vi "DWE Decode Data.vi"(8 "Errors In":T1, 9 "Prev time stamp":timestamp, 10 "Time Stamp":timestamp, 11 "Data Array":string[](array[string])) -> (0 "Errors Out":T1, 3 "logData Out":T2)   [LabVIEW 2014]
doc: "Decode hex data obtained from inverter boards into decimal measurements. DC bus voltage, current RMS, motor power, temp."
uses:
  TypeDefs/DWE Errors.ctl
panel:
  out "Elapsed time (min)":dbl
  out "Elapsed time (sec)":dbl
  in  "logData In":T3
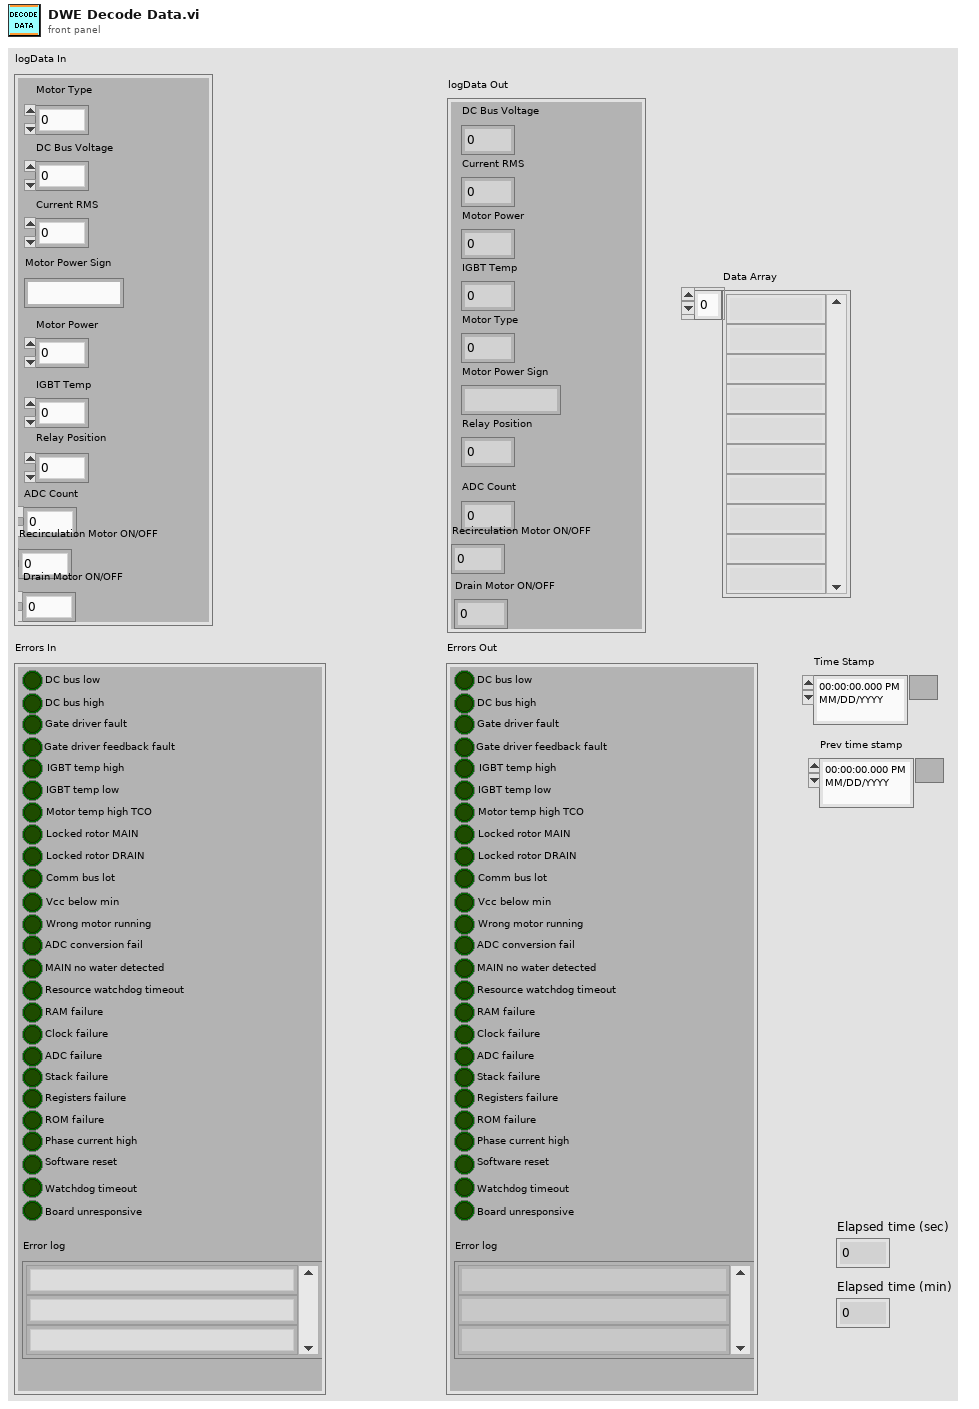
[diagram p1: front panel]
types:
  T1 = typedef "DWE Errors.ctl" = cluster{"DC bus low":bool, "DC bus high":bool, "Gate driver fault":bool, "Gate driver feedback fault":bool, "IGBT temp high":bool, "IGBT temp low":bool, "Motor temp high TCO":bool, "Locked rotor MAIN":bool, "Locked rotor DRAIN":bool, "Comm bus lot":bool, "Vcc below min":bool, "Wrong motor running":bool, "ADC conversion fail":bool, "MAIN no water detected":bool, "Resource watchdog timeout":bool, "RAM failure":bool, "Clock failure":bool, "ADC failure":bool, "Stack failure":bool, "Registers failure":bool, "ROM failure":bool, "Phase current high":bool, "Software reset":bool, "Watchdog timeout":bool, "Error log":string[], "Board unresponsive":bool}
  T2 = cluster{"DC Bus Voltage":dbl, "Current RMS":dbl, "Motor Power":dbl, "IGBT Temp":u16, "Motor Type":u16, "Motor Power Sign":string, "Relay Position":u16, "ADC Count":dbl, "Recirculation Motor ON/OFF":u16, "Drain Motor ON/OFF":u16}
  T3 = cluster{"DC Bus Voltage":dbl, "Current RMS":dbl, "Motor Power":dbl, "IGBT Temp":u32, "Motor Type":u16, "Motor Power Sign":string, "Relay Position":u16, "ADC Count":dbl, "Recirculation Motor ON/OFF":u32, "Drain Motor ON/OFF":u16}
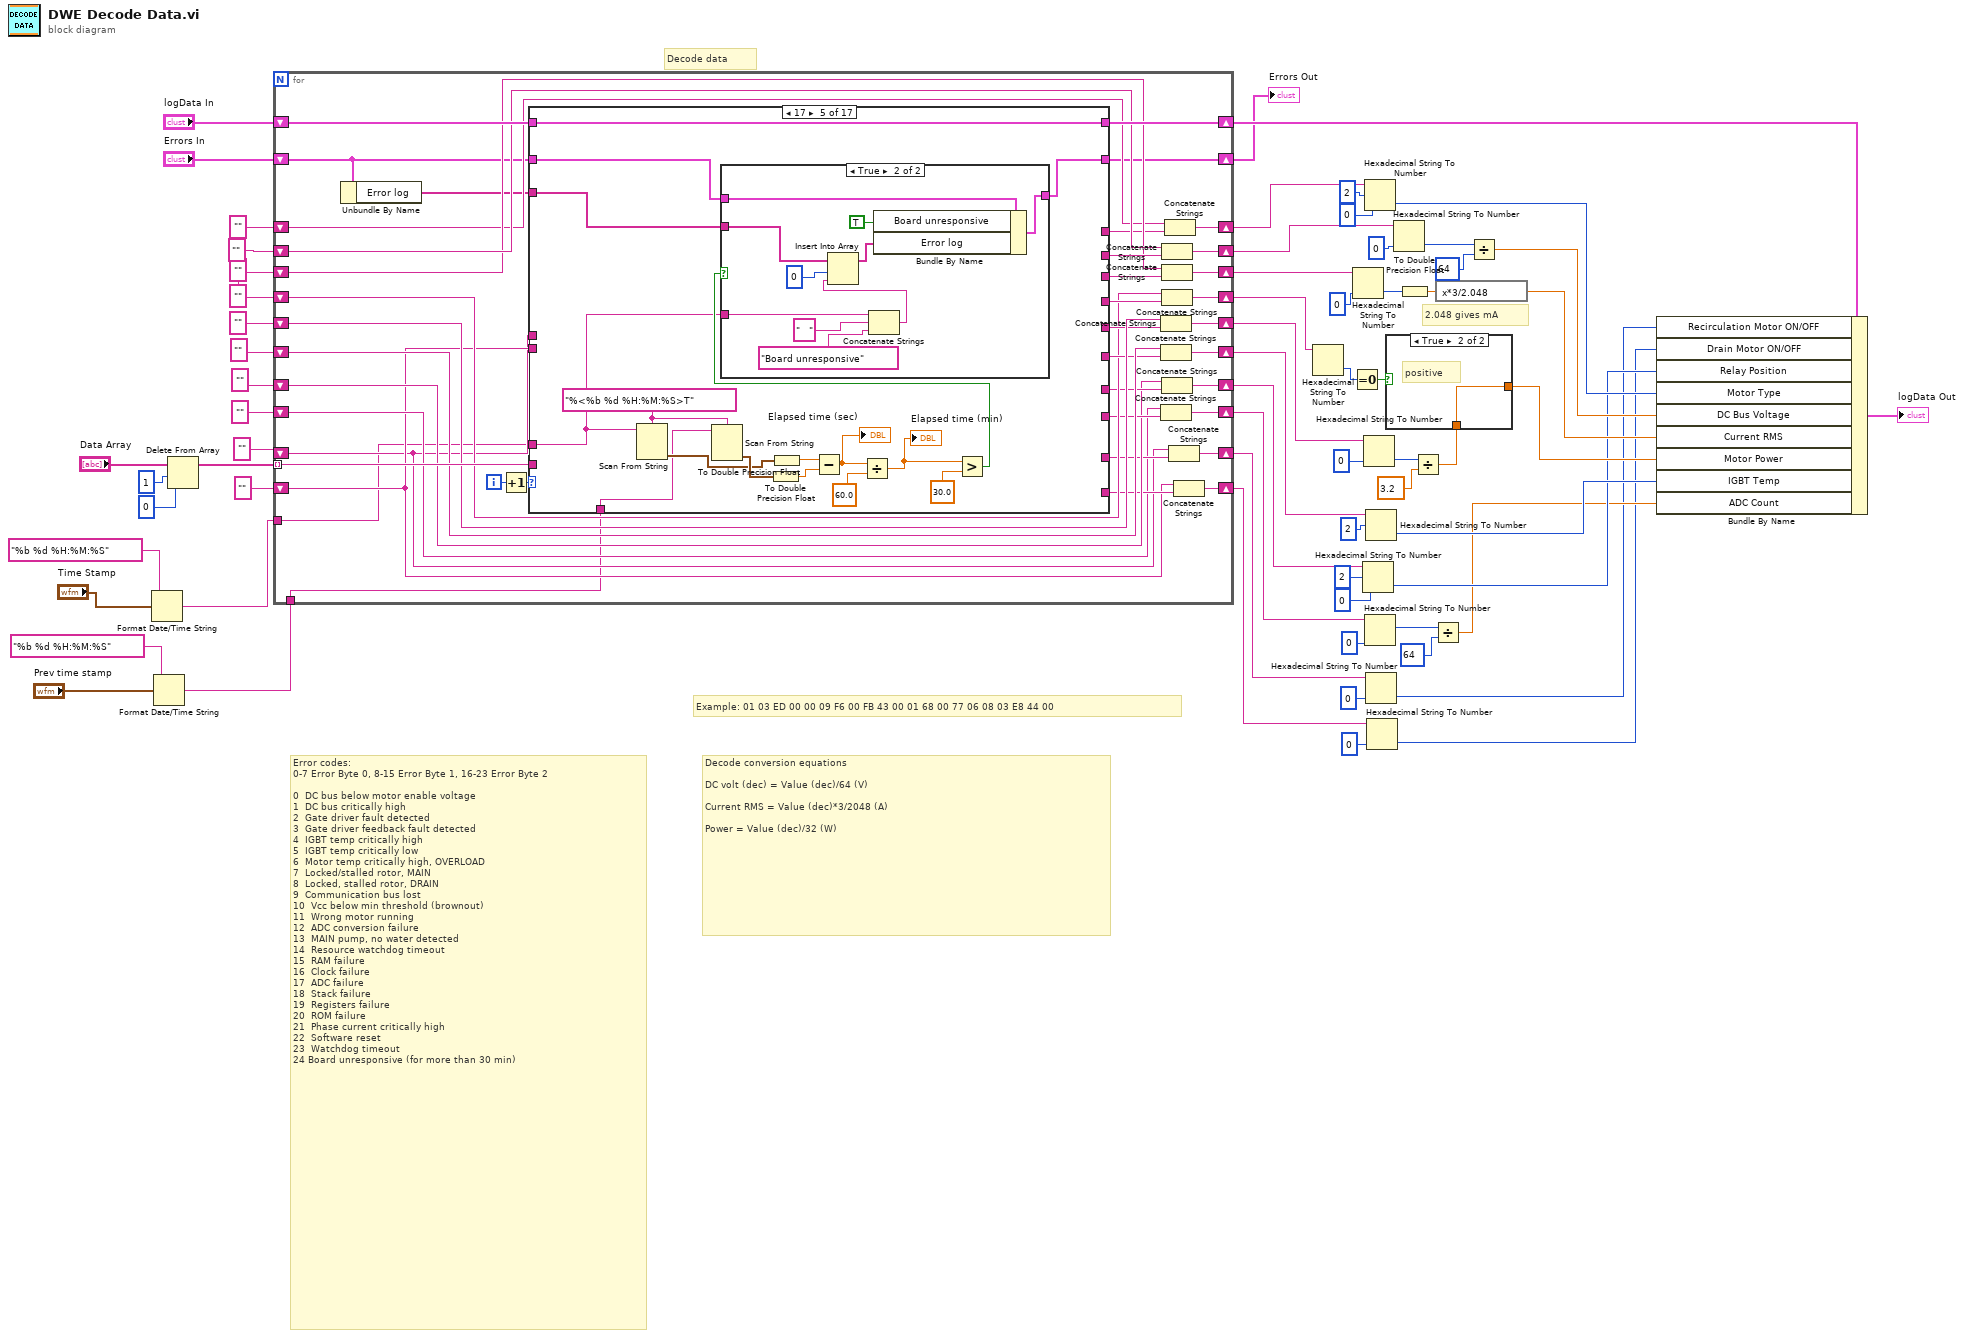
[diagram p0: block diagram]
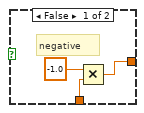
[diagram p2: hidden frame]
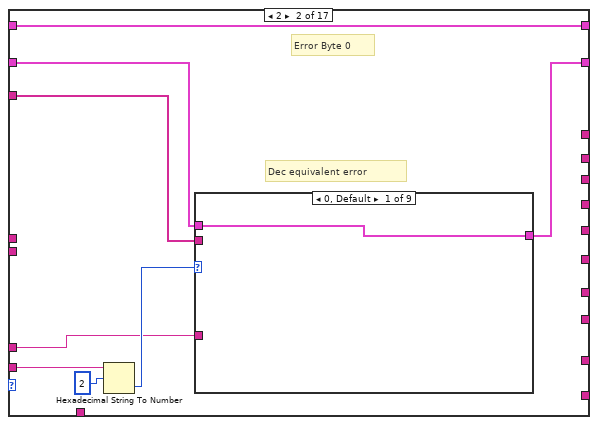
[diagram p4: hidden frame]
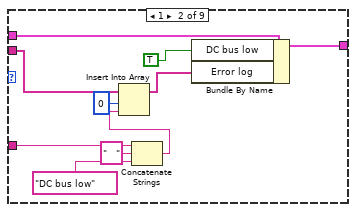
[diagram p5: hidden frame]
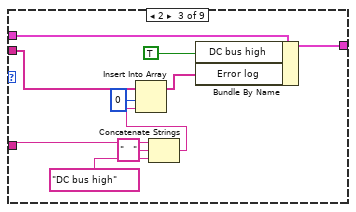
[diagram p6: hidden frame]
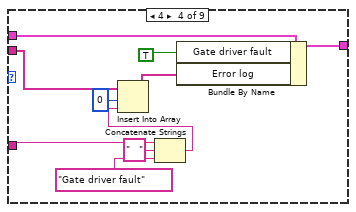
[diagram p7: hidden frame]
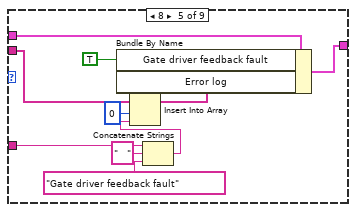
[diagram p8: hidden frame]
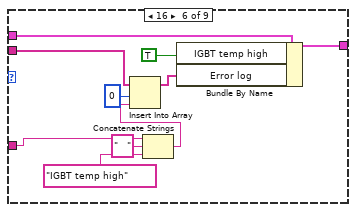
[diagram p9: hidden frame]
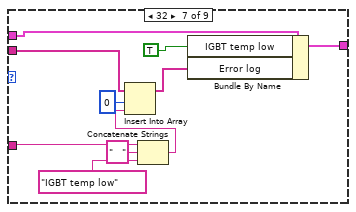
[diagram p10: hidden frame]
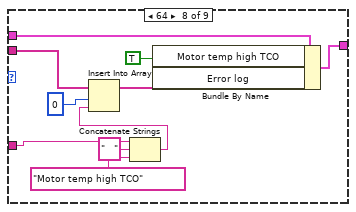
[diagram p11: hidden frame]
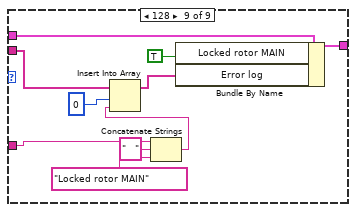
[diagram p12: hidden frame]
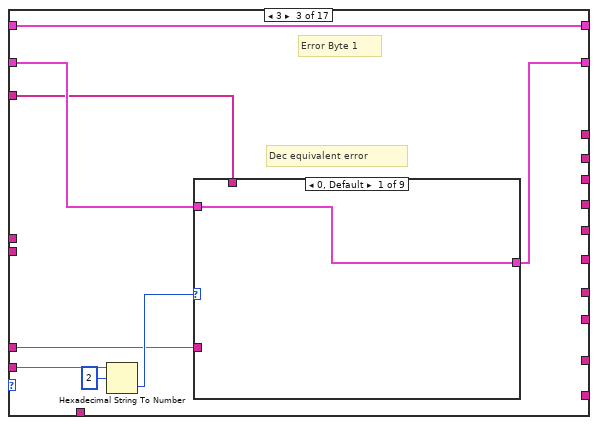
[diagram p13: hidden frame]
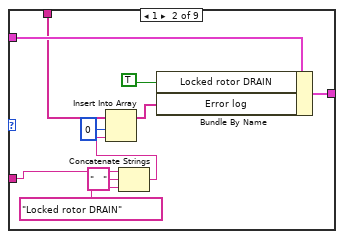
[diagram p14: hidden frame]
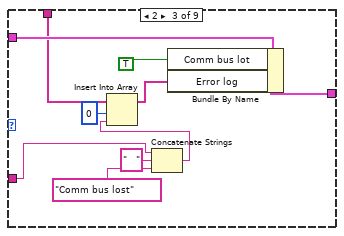
[diagram p15: hidden frame]
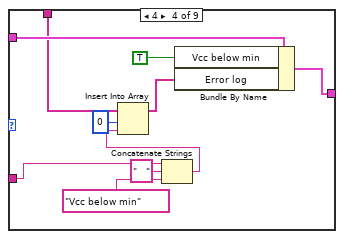
[diagram p16: hidden frame]
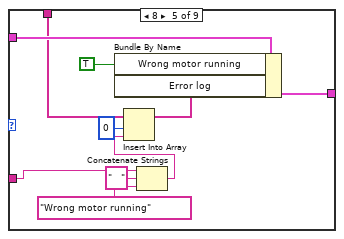
[diagram p17: hidden frame]
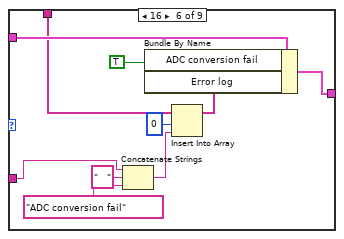
[diagram p18: hidden frame]
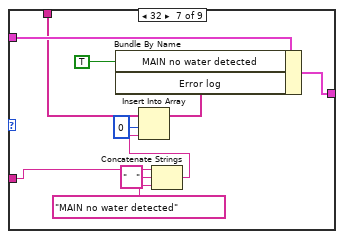
[diagram p19: hidden frame]
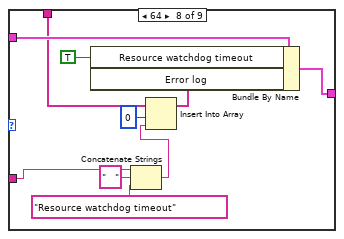
[diagram p20: hidden frame]
diagram:
  # "2.048 gives mA"
  # "Decode conversion equations\n\nDC volt (dec) = Value (dec)/64 (V)\n\nCurrent RMS = Value (dec)*3/2048 (A)\n\nPower = Value (dec)/32 (W)"
  # "Error codes:\n0-7 Error Byte 0, 8-15 Error Byte 1, 16-23 Error Byte 2\n\n0  DC bus below motor enable voltage\n1  DC bus critically high\n2  Gate driver fault detected\n3  Gate driver feedback fault detected\n4  IGBT temp critically high\n5  IGBT temp critically low\n6  Motor temp critically high, OVERLOAD\n7  Locked/stalled rotor, MAIN\n8  Locked, stalled rotor, DRAIN\n9  Communication bus lost\n10  Vcc below min threshold (brownout)\n11  Wrong motor running\n12  ADC conversion failure\n13  MAIN pump, no water detected\n14  Resource watchdog timeout\n15  RAM failure \n16  Clock failure\n17  ADC failure\n18  Stack failure\n19  Registers failure\n20  ROM failure\n21  Phase current critically high\n22  Software reset\n23  Watchdog timeout\n24 Board unresponsive (for more than 30 min)"
  # "Example: 01 03 ED 00 00 09 F6 00 FB 43 00 01 68 00 77 06 08 03 E8 44 00"
  # "Decode data"
  n1 = Format Date/Time String(time format string (%c)="%b %d %H:%M:%S", seconds (now)="Time Stamp") -> (date/time string=w4:string)  [unwired: 1 in]
  n2 = Format Date/Time String(time format string (%c)="%b %d %H:%M:%S", seconds (now)="Prev time stamp") -> (date/time string=w1:string)  [unwired: 1 in]
  n3 = Delete From Array(array="Data Array", length=1, index=0) -> (array with subset deleted=w7:string[])  [unwired: 1 out]
  n4 = for {
    tunnel: w7 -> [w106] mode=indexing
    shift-right: [w104] -> w55
    shift-left: "logData In" -> [w103]
    shift-right: [w99] -> w57
    shift-left: "" -> [w101]
    shift-right: [w96] -> w61
    shift-left: "" -> [w98]
    shift-right: [w93] -> w64
    shift-left: "" -> [w95]
    shift-right: [w90] -> w66
    shift-left: "" -> [w92]
    shift-right: [w87] -> w41
    shift-left: "" -> [w88]
    shift-right: [w85] -> w35
    shift-left: "" -> [w83]
    shift-right: [w86] -> w40
    shift-left: "Errors In" -> [w70]
    shift-right: [w82] -> w29
    shift-left: "" -> [w78]
    shift-right: [w79] -> w23
    shift-left: "" -> [w73]
    shift-right: [w76] -> w18
    shift-left: "" -> [w71]
    shift-right: [w77] -> w17
    shift-left: "" -> [w72]
    tunnel: w4 -> [w68]
    tunnel: w1 -> [w67]
    i -> [w105]
    n5 = Unbundle By Name(w70) -> ("Error log"=w69:string[])
    n6 = Increment(x=w105) -> (x+1=w102:i32)
    n7 = case shown="17" w102 {
      tunnel: w106 -> [w108 w117 w206 w294 _ w407 w411 w415 w420 w425 w431 w435 w440 w442 w446 w451 w460]
      tunnel: w103 -> [w109 w112 w202 w291 w392 w408 w413 w418 w423 w428 w433 w438 w441 w444 w449 w454 w464]
      tunnel: [w109 w112 w202 w291 w392 w408 w413 w418 w423 w428 w433 w438 w441 w444 w449 w454 w464] -> w104
      tunnel: [_ _ _ _ _ w406 w410 _ _ _ _ _ _ _ _ _ _] -> w100
      tunnel: [_ _ _ _ _ _ _ w416 w421 _ _ _ _ _ _ _ _] -> w97
      tunnel: [_ _ _ _ _ _ _ _ _ _ w429 w436 _ _ _ _ _] -> w94
      tunnel: [_ _ _ _ _ _ _ _ _ _ _ _ w440 _ _ _ _] -> w91
      tunnel: [w108 _ _ _ _ _ _ _ _ _ _ _ _ _ _ _ _] -> w89
      tunnel: w70 -> [w107 w114 w203 w292 w391 w404 w409 w414 w419 w427 w430 w434 w439 w443 w448 w453 w463]
      tunnel: [w107 w113 w201 w290 w389 w404 w409 w414 w419 w427 w430 w434 w439 w443 w448 w453 w463] -> w86
      tunnel: [_ _ _ _ _ _ _ _ _ w424 _ _ _ _ _ _ _] -> w84
      tunnel: [_ _ _ _ _ _ _ _ _ _ _ _ _ w442 _ _ _] -> w81
      tunnel: [_ _ _ _ _ _ _ _ _ _ _ _ _ _ w445 w450 _] -> w80
      tunnel: [_ _ _ _ _ _ _ _ _ _ _ _ _ _ _ _ w458] -> w74
      tunnel: [_ _ _ _ _ _ _ _ _ _ _ _ _ _ _ _ w457] -> w75
      tunnel: w71 -> [_ _ _ _ _ _ _ _ _ _ _ _ _ _ _ _ w456]
      tunnel: w72 -> [_ _ _ _ _ _ _ _ _ _ _ _ _ _ _ _ w455]
      tunnel: w69 -> [_ w110 w200 w288 w390 _ _ _ _ _ _ _ _ _ _ _ _]
      tunnel: w68 -> [_ w111 w199 w289 w377 _ _ _ _ _ _ _ _ _ _ _ _]
      tunnel: w67 -> [_ _ _ _ w382 _ _ _ _ _ _ _ _ _ _ _ _]
      frame 1, Default {
        # "Motor type"
      }
      frame 2 {
        # "Dec equivalent error"
        # "Error Byte 0"
        n8 = Hexadecimal String To Number(string=w117, offset=2) -> (number=w115:u32)  [unwired: 1 in, 1 out]
        n9 = case shown="0, Default" w115 {
          tunnel: w114 -> [w118 w126 w138 w148 w157 w167 w177 w187 w197]
          tunnel: [w118 w127 w137 w147 w156 w166 w176 w186 w196] -> w113
          tunnel: w111 -> [_ w122 w132 w142 w152 w162 w172 w182 w192]
          tunnel: w110 -> [_ w121 w131 w141 w151 w161 w170 w180 w191]
          frame 0, Default {
          }
          frame 1 {
            n10 = Concatenate Strings(w122, "   " ("string"), "DC bus low") -> (w125:string)
            n11 = Insert Into Array(array=w121, index=0, new element=w125) -> (w120:string[])
            n12 = Bundle By Name(cluster=w126, "DC bus low"=TRUE, "Error log"=w120) -> (w127:T1)
          }
          frame 2 {
            n13 = Concatenate Strings(w132, "   " ("string"), "DC bus high") -> (w135:string)
            n14 = Insert Into Array(array=w131, index=0, new element=w135) -> (w130:string[])
            n15 = Bundle By Name(cluster=w138, "DC bus high"=TRUE ("Errors.Locked rotor DRAIN"), "Error log"=w130) -> (w137:T1)
          }
          frame 4 {
            n16 = Concatenate Strings(w142, "   " ("string"), "Gate driver fault") -> (w145:string)
            n17 = Insert Into Array(array=w141, index=0, new element=w145) -> (w140:string[])
            n18 = Bundle By Name(cluster=w148, "Gate driver fault"=TRUE ("Errors.Vcc below min"), "Error log"=w140) -> (w147:T1)
          }
          frame 8 {
            n19 = Concatenate Strings(w152, "   " ("string"), "Gate driver feedback fault") -> (w155:string)
            n20 = Insert Into Array(array=w151, index=0, new element=w155) -> (w150:string[])
            n21 = Bundle By Name(cluster=w157, "Gate driver feedback fault"=TRUE ("Errors.Vcc below min"), "Error log"=w150) -> (w156:T1)
          }
          frame 16 {
            n22 = Concatenate Strings(w162, "   " ("string"), "IGBT temp high") -> (w165:string)
            n23 = Insert Into Array(array=w161, index=0, new element=w165) -> (w160:string[])
            n24 = Bundle By Name(cluster=w167, "IGBT temp high"=TRUE ("Errors.Vcc below min"), "Error log"=w160) -> (w166:T1)
          }
          frame 32 {
            n25 = Concatenate Strings(w172, "   " ("string"), "IGBT temp low") -> (w175:string)
            n26 = Insert Into Array(array=w170, index=0, new element=w175) -> (w171:string[])
            n27 = Bundle By Name(cluster=w177, "IGBT temp low"=TRUE ("Errors.Vcc below min"), "Error log"=w171) -> (w176:T1)
          }
          frame 64 {
            n28 = Concatenate Strings(w182, "   " ("string"), "Motor temp high TCO") -> (w185:string)
            n29 = Insert Into Array(array=w180, index=0, new element=w185) -> (w181:string[])
            n30 = Bundle By Name(cluster=w187, "Motor temp high TCO"=TRUE ("Errors.Vcc below min"), "Error log"=w181) -> (w186:T1)
          }
          frame 128 {
            n31 = Concatenate Strings(w192, "   " ("string"), "Locked rotor MAIN") -> (w190:string)
            n32 = Insert Into Array(array=w191, index=0, new element=w190) -> (w189:string[])
            n33 = Bundle By Name(cluster=w197, "Locked rotor MAIN"=TRUE ("Errors.Vcc below min"), "Error log"=w189) -> (w196:T1)
          }
        }
      }
      frame 3 {
        # "Dec equivalent error"
        # "Error Byte 1"
        n34 = Hexadecimal String To Number(string=w206, offset=2) -> (number=w204:u32)  [unwired: 1 in, 1 out]
        n35 = case shown="0, Default" w204 {
          tunnel: w203 -> [w207 w215 w227 w237 w246 w256 w266 w276 w286]
          tunnel: [w207 w216 w226 w236 w245 w255 w265 w275 w285] -> w201
          tunnel: w200 -> [_ w213 w220 w230 w239 w250 w260 w270 w280]
          tunnel: w199 -> [_ w212 w221 w231 w241 w251 w261 w271 w281]
          frame 0, Default {
          }
          frame 1 {
            n36 = Concatenate Strings(w212, "   " ("string"), "Locked rotor DRAIN") -> (w211:string)
            n37 = Insert Into Array(array=w213, index=0, new element=w211) -> (w214:string[])
            n38 = Bundle By Name(cluster=w215, "Locked rotor DRAIN"=TRUE ("DC bus low"), "Error log"=w214) -> (w216:T1)
          }
          frame 2 {
            n39 = Concatenate Strings(w221, "   " ("string"), "Comm bus lost") -> (w224:string)
            n40 = Insert Into Array(array=w220, index=0, new element=w224) -> (w219:string[])
            n41 = Bundle By Name(cluster=w227, "Comm bus lot"=TRUE ("Errors.Locked rotor DRAIN"), "Error log"=w219) -> (w226:T1)
          }
          frame 4 {
            n42 = Concatenate Strings(w231, "   " ("string"), "Vcc below min") -> (w234:string)
            n43 = Insert Into Array(array=w230, index=0, new element=w234) -> (w229:string[])
            n44 = Bundle By Name(cluster=w237, "Vcc below min"=TRUE ("Errors.Vcc below min"), "Error log"=w229) -> (w236:T1)
          }
          frame 8 {
            n45 = Concatenate Strings(w241, "   " ("string"), "Wrong motor running") -> (w244:string)
            n46 = Insert Into Array(array=w239, index=0, new element=w244) -> (w240:string[])
            n47 = Bundle By Name(cluster=w246, "Wrong motor running"=TRUE ("Errors.Vcc below min"), "Error log"=w240) -> (w245:T1)
          }
          frame 16 {
            n48 = Concatenate Strings(w251, "   " ("string"), "ADC conversion fail") -> (w254:string)
            n49 = Insert Into Array(array=w250, index=0, new element=w254) -> (w249:string[])
            n50 = Bundle By Name(cluster=w256, "ADC conversion fail"=TRUE ("Errors.Vcc below min"), "Error log"=w249) -> (w255:T1)
          }
          frame 32 {
            n51 = Concatenate Strings(w261, "   " ("string"), "MAIN no water detected") -> (w264:string)
            n52 = Insert Into Array(array=w260, index=0, new element=w264) -> (w259:string[])
            n53 = Bundle By Name(cluster=w266, "MAIN no water detected"=TRUE ("Errors.Vcc below min"), "Error log"=w259) -> (w265:T1)
          }
          frame 64 {
            n54 = Concatenate Strings(w271, "   " ("string"), "Resource watchdog timeout") -> (w274:string)
            n55 = Insert Into Array(array=w270, index=0, new element=w274) -> (w269:string[])
            n56 = Bundle By Name(cluster=w276, "Resource watchdog timeout"=TRUE ("Errors.Vcc below min"), "Error log"=w269) -> (w275:T1)
          }
          frame 128 {
            n57 = Concatenate Strings(w281, "   " ("string"), "RAM failure") -> (w284:string)
            n58 = Insert Into Array(array=w280, index=0, new element=w284) -> (w279:string[])
            n59 = Bundle By Name(cluster=w286, "RAM failure"=TRUE ("Errors.Vcc below min"), "Error log"=w279) -> (w285:T1)
          }
        }
      }
      frame 4 {
        # "Error Byte 2"
        # "Dec equivalent error"
        n60 = Hexadecimal String To Number(string=w294, offset=2) -> (number=w293:u32)  [unwired: 1 in, 1 out]
        n61 = case shown="0, Default" w293 {
          tunnel: w292 -> [w296 w304 w316 w326 w335 w345 w355 w365 w375]
          tunnel: [w296 w305 w315 w325 w334 w344 w354 w364 w374] -> w290
          tunnel: w289 -> [_ w299 w309 w319 w329 w339 w349 w359 w369]
          tunnel: w288 -> [_ w298 w308 w318 w328 w338 w348 w358 w368]
          frame 0, Default {
          }
          frame 1 {
            n62 = Concatenate Strings(w299, "   " ("string"), "Clock failure") -> (w300:string)
            n63 = Insert Into Array(array=w298, index=0, new element=w300) -> (w297:string[])
            n64 = Bundle By Name(cluster=w304, "Clock failure"=TRUE ("DC bus low"), "Error log"=w297) -> (w305:T1)
          }
          frame 2 {
            n65 = Concatenate Strings(w309, "   " ("string"), "ADC failure") -> (w310:string)
            n66 = Insert Into Array(array=w308, index=0, new element=w310) -> (w307:string[])
            n67 = Bundle By Name(cluster=w316, "ADC failure"=TRUE ("Errors.Locked rotor DRAIN"), "Error log"=w307) -> (w315:T1)
          }
          frame 4 {
            n68 = Concatenate Strings(w319, "   " ("string"), "Stack failure") -> (w320:string)
            n69 = Insert Into Array(array=w318, index=0, new element=w320) -> (w317:string[])
            n70 = Bundle By Name(cluster=w326, "Stack failure"=TRUE ("Errors.Vcc below min"), "Error log"=w317) -> (w325:T1)
          }
          frame 8 {
            n71 = Concatenate Strings(w329, "   " ("string"), "Registers failure") -> (w330:string)
            n72 = Insert Into Array(array=w328, index=0, new element=w330) -> (w327:string[])
            n73 = Bundle By Name(cluster=w335, "Registers failure"=TRUE ("Errors.Vcc below min"), "Error log"=w327) -> (w334:T1)
          }
          frame 16 {
            n74 = Concatenate Strings(w339, "   " ("string"), "ROM failure") -> (w340:string)
            n75 = Insert Into Array(array=w338, index=0, new element=w340) -> (w337:string[])
            n76 = Bundle By Name(cluster=w345, "ROM failure"=TRUE ("Errors.Vcc below min"), "Error log"=w337) -> (w344:T1)
          }
          frame 32 {
            n77 = Concatenate Strings(w349, "   " ("string"), "Phase current high") -> (w350:string)
            n78 = Insert Into Array(array=w348, index=0, new element=w350) -> (w347:string[])
            n79 = Bundle By Name(cluster=w355, "Phase current high"=TRUE ("Errors.Vcc below min"), "Error log"=w347) -> (w354:T1)
          }
          frame 64 {
            n80 = Concatenate Strings(w359, "   " ("string"), "Software reset") -> (w360:string)
            n81 = Insert Into Array(array=w358, index=0, new element=w360) -> (w357:string[])
            n82 = Bundle By Name(cluster=w365, "Software reset"=TRUE ("Errors.Vcc below min"), "Error log"=w357) -> (w364:T1)
          }
          frame 128 {
            n83 = Concatenate Strings(w369, "   " ("string"), "Watchdog timeout") -> (w370:string)
            n84 = Insert Into Array(array=w368, index=0, new element=w370) -> (w367:string[])
            n85 = Bundle By Name(cluster=w375, "Watchdog timeout"=TRUE ("Errors.Vcc below min"), "Error log"=w367) -> (w374:T1)
          }
        }
      }
      frame 17 {
        w378 = "%<%b %d %H:%M:%S>T" ("format string")
        n86 = Scan From String(format string=w378, input string=w377) -> (output 1=w383:timestamp)  [unwired: 3 in, 3 out]
        n87 = Scan From String(format string=w378, input string=w382) -> (output 1=w385:timestamp)  [unwired: 3 in, 3 out]
        n88 = To Double Precision Float(number=w385) -> (double precision float=w386:dbl)
        n89 = To Double Precision Float(number=w383) -> (double precision float=w384:dbl)
        n90 = Subtract(x=w384, y=w386) -> (x-y=w388:dbl)
        "Elapsed time (sec)" <- w388
        n91 = Divide(x=w388, y=60.0) -> (x/y=w381:dbl)
        "Elapsed time (min)" <- w381
        n92 = Greater?(x=w381, y=30.0) -> (0:w379:bool)
        n93 = case shown="True" w379 {
          tunnel: w391 -> [w393 w401]
          tunnel: [w393 w402] -> w389
          tunnel: w377 -> [_ w396]
          tunnel: w390 -> [_ w395]
          frame False {
          }
          frame True {
            n94 = Concatenate Strings(w396, "   " ("string"), "Board unresponsive") -> (w397:string)
            n95 = Insert Into Array(array=w395, index=0, new element=w397) -> (w394:string[])
            n96 = Bundle By Name(cluster=w401, "Board unresponsive"=TRUE ("DC bus low"), "Error log"=w394) -> (w402:T1)
          }
        }
      }
      frame 5 {
        # "DC Bus Voltage MSB"
        n97 = String Subset(string=w407, offset (0)=2) -> (substring=w406:string)  [unwired: 1 in]
      }
      frame 6 {
        # "DC Bus Voltage LSB"
        n98 = String Subset(string=w411, offset (0)=2) -> (substring=w410:string)  [unwired: 1 in]
      }
      frame 7 {
        # "Current RMS MSB"
        n99 = String Subset(string=w415, offset (0)=2) -> (substring=w416:string)  [unwired: 1 in]
      }
      frame 8 {
        # "Current RMS LSB"
        n100 = String Subset(string=w420, offset (0)=2) -> (substring=w421:string)  [unwired: 1 in]
      }
      frame 9 {
        # "0x00 positive\n0x01 negative"
        # "Motor Power Sign"
        n101 = String Subset(string=w425, offset (0)=2) -> (substring=w424:string)  [unwired: 1 in]
      }
      frame 10 {
        # "Motor Power MSB"
        n102 = String Subset(string=w431, offset (0)=2) -> (substring=w429:string)  [unwired: 1 in]
      }
      frame 11 {
        # "Motor Power LSB"
        n103 = String Subset(string=w435, offset (0)=2) -> (substring=w436:string)  [unwired: 1 in]
      }
      frame 12 {
        # "IGBT Temp"
      }
      frame 13 {
        # "Relay Position State"
      }
      frame 14 {
        # "Relay Position ADC Count MSB"
        n104 = String Subset(string=w446, offset (0)=2) -> (substring=w445:string)  [unwired: 1 in]
      }
      frame 15 {
        # "Relay Position ADC Count LSB"
        n105 = String Subset(string=w451, offset (0)=2) -> (substring=w450:string)  [unwired: 1 in]
      }
      frame 16 {
        # "ALT Test Profile Index"
        n106 = Hexadecimal String To Number(string=w460, offset=2, default (0uL)=u32 0 ("default (0 U32)")) -> (number=w459:u32)  [unwired: 1 out]
        n107 = case shown="2, 6, 10, 14, 18, 22, 26" w459 {
          tunnel: [w465 w467 "01" "00"] -> w458
          tunnel: w455 -> [w465 w467 _ _]
          tunnel: w456 -> [_ _ w469 w471]
          tunnel: ["01" "00" w469 w471] -> w457
          frame 0, 4, 8, 12, 16, 20, 24, 28, Default {
            # "Recirculation motor ON"
          }
          frame 1, 5, 9, 13, 17, 21, 25, 29 {
            # "Recirculation motor OFF"
          }
          frame 2, 6, 10, 14, 18, 22, 26 {
            # "drain motor ON"
          }
          frame 3, 7, 11, 15, 19, 23, 27 {
            # "drain motor OFF"
          }
        }
      }
    }
    n108 = Concatenate Strings(w95, w94) -> (w93:string)
    n109 = Concatenate Strings(w92, w91) -> (w90:string)
    n110 = Concatenate Strings(w73, w80) -> (w79:string)
    n111 = Concatenate Strings(w101, w100) -> (w99:string)
    n112 = Concatenate Strings(w98, w97) -> (w96:string)
    n113 = Concatenate Strings(w83, w84) -> (w85:string)
    n114 = Concatenate Strings(w78, w81) -> (w82:string)
    n115 = Concatenate Strings(w88, w89) -> (w87:string)
    n116 = Concatenate Strings(w71, w75) -> (w76:string)
    n117 = Concatenate Strings(w72, w74) -> (w77:string)
  }
  "Errors Out" <- w40
  n118 = Hexadecimal String To Number(string=w35) -> (number=w36:u32)  [unwired: 2 in, 1 out]
  n119 = Equal To 0?(x=w36) -> (x = 0?=w34:bool)
  n120 = Hexadecimal String To Number(string=w61, default (0uL)=u16 0 ("default (0 U32)")) -> (number=w38:u16)  [unwired: 1 in, 1 out]
  n121 = Hexadecimal String To Number(string=w29, offset=2, default (0uL)=u32 0 ("default (0 U32)")) -> (number=w28:u32)  [unwired: 1 out]
  n122 = Hexadecimal String To Number(string=w64, default (0uL)=u16 0 ("default (0 U32)")) -> (number=w53:u16)  [unwired: 1 in, 1 out]
  n123 = Hexadecimal String To Number(string=w41, offset=2, default (0uL)=u32 0 ("default (0 U32)")) -> (number=w42:u32)  [unwired: 1 out]
  n124 = Hexadecimal String To Number(string=w23, default (0uL)=u16 0 ("default (0 U32)")) -> (number=w24:u16)  [unwired: 1 in, 1 out]
  n125 = Hexadecimal String To Number(string=w66, offset=2) -> (number=w43:u32)  [unwired: 1 in, 1 out]
  n126 = Hexadecimal String To Number(string=w18, default (0uL)=u32 0 ("default (0 U32)")) -> (number=w16:u32)  [unwired: 1 in, 1 out]
  n127 = Hexadecimal String To Number(string=w17, default (0uL)=u32 0 ("default (0 U32)")) -> (number=w15:u32)  [unwired: 1 in, 1 out]
  n128 = Hexadecimal String To Number(string=w57, default (0uL)=u16 0 ("default (0 U32)")) -> (number=w52:u16)  [unwired: 1 in, 1 out]
  n129 = To Double Precision Float(number=w38) -> (double precision float=w50:dbl)
  n130 = Divide(x=w53, y=3.2) -> (x/y=w13:dbl)
  n131 = case shown="True" w34 {
    tunnel: w13 -> [w474 w476]
    tunnel: [w473 w476] -> w39
    frame False {
      # "negative"
      n132 = Multiply(x=-1.0, y=w474) -> (x*y=w473:dbl)
    }
    frame True {
      # "positive"
    }
  }
  n133 = Divide(x=w24, y=u16 64) -> (x/y=w22:dbl)
  n134 = expression code="x*3/2.048"(w50) -> (w48:dbl)
  n135 = Divide(x=w52, y=u16 64) -> (x/y=w49:dbl)
  n136 = Bundle By Name(cluster=w55, "Recirculation Motor ON/OFF"=w16, "Drain Motor ON/OFF"=w15, "Relay Position"=w28, "Motor Type"=w42, "DC Bus Voltage"=w49, "Current RMS"=w48, "Motor Power"=w39, "IGBT Temp"=w43, "ADC Count"=w22) -> (→"logData Out":T3)
